vi "MESADCSubmitTestData.vi"(1 "MES_info":T1={"工号"="2300013", "站别"="F1", "站名"="写信息", "表名称"="test", "工单号"="85255", "条码"="EC82637770B0", "路径"="", "是否连接"="", "电脑名"=""}, 5 "错误输入（无错误）":errorcluster) -> (14 "result 2":i32, 15 "message":string, 17 "布尔":bool, 19 "错误输出":errorcluster)   [LabVIEW 2014]
uses:
  MES.ctl
  MESControldll.dll
panel:
  out "errbuf":string
  out "m_paramAVal":string
  out "PointGroup 2":string
  out "PointName 2":string
  out "userid 2":string
  out "POnum 1":i32
  out "result":i32
  # "2300013"
  # "1001594"
  # "0是代表OK，-1代表NG"
  # "1001608"
  # "447BBBCDFA60"
  # "447BBBA1A0D0"
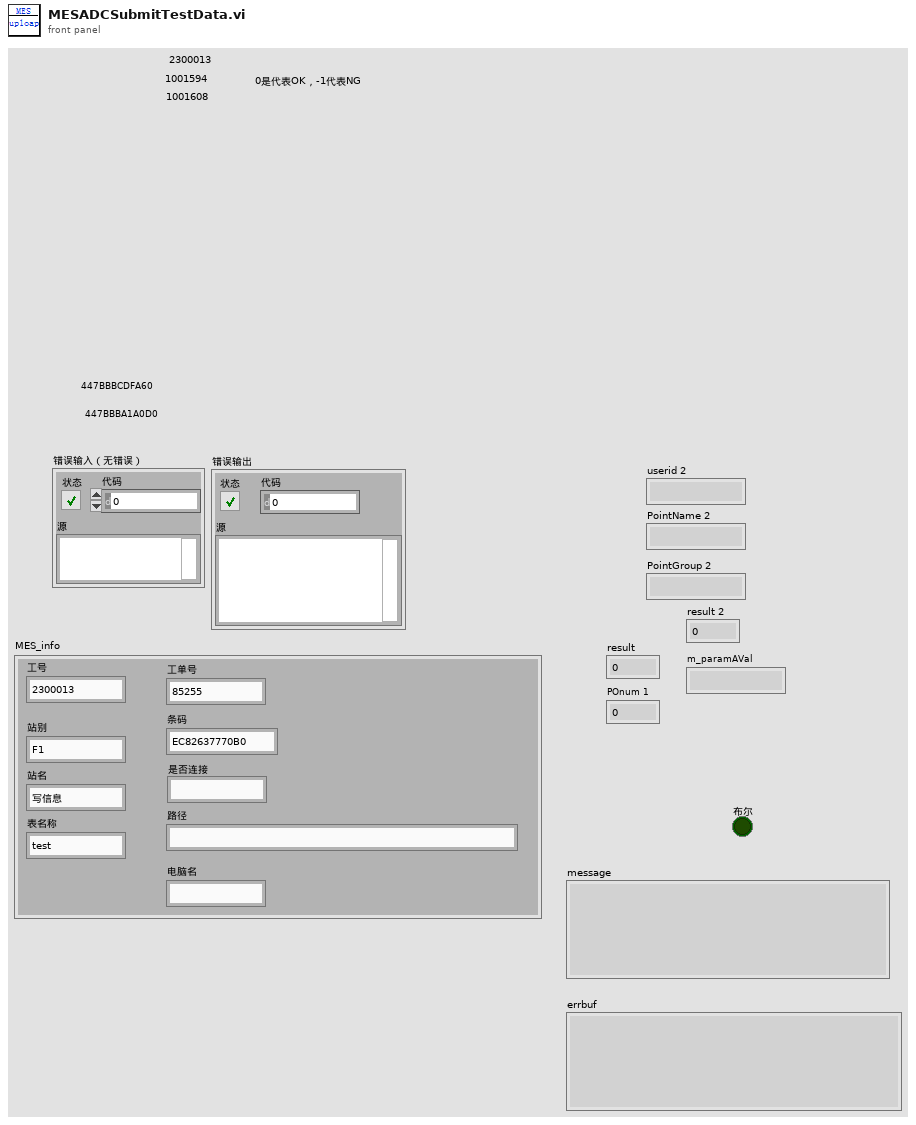
[diagram p1: front panel]
types:
  T1 = typedef "MES.ctl" = cluster{"工号":string, "站别":string, "站名":string, "表名称":string, "工单号":string, "条码":string, "路径":string, "是否连接":string, "电脑名":string}
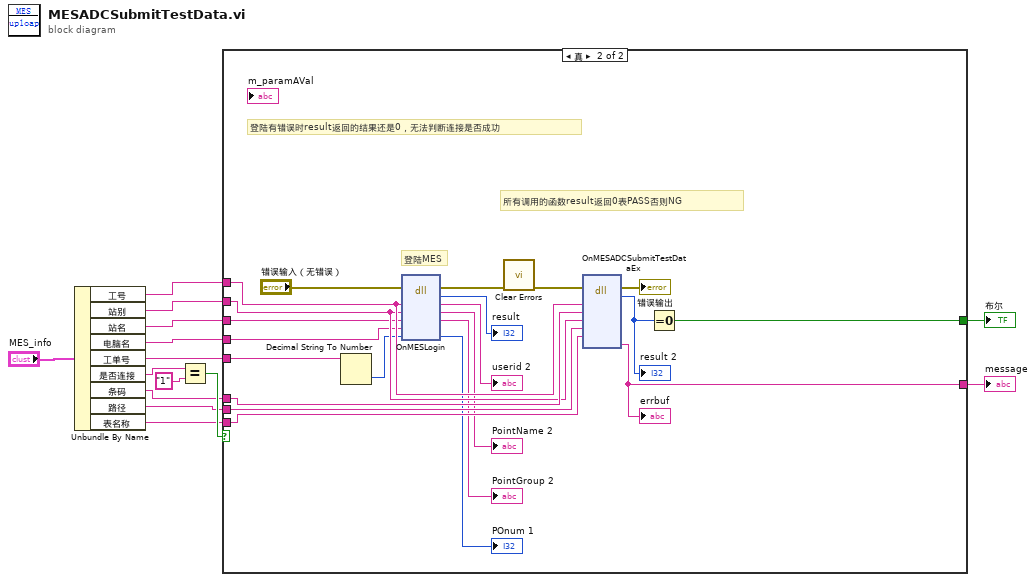
[diagram p0: block diagram]
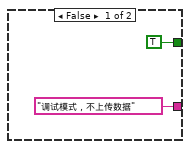
[diagram p2: hidden frame]
diagram:
  n1 = Unbundle By Name("MES_info") -> ("工号"=w1:string, "站别"=w10:string, "站名"=w9:string, "电脑名"=w8:string, "工单号"=w7:string, "是否连接"=w3:string, "条码"=w4:string, "路径"=w5:string, "表名称"=w6:string)
  n2 = Equal?(x=w3, y="1") -> (x = y?=w12:bool)
  n3 = case shown="真" w12 {
    tunnel: [TRUE w37] -> w14
    tunnel: ["调试模式，不上传数据" w36] -> w13
    tunnel: w1 -> [_ w35]
    tunnel: w4 -> [_ w34]
    tunnel: w10 -> [_ w33]
    tunnel: w7 -> [_ w32]
    tunnel: w6 -> [_ w31]
    tunnel: w9 -> [_ w30]
    tunnel: w8 -> [_ w29]
    tunnel: w5 -> [_ w28]
    frame False {
    }
    frame True {
      # "登陆MES"
      # "登陆有错误时result返回的结果还是0，无法判断连接是否成功"
      # "所有调用的函数result返回0表PASS否则NG"
      n4 = Decimal String To Number(string=w32) -> (number=w21:i32)  [unwired: 2 in, 1 out]
      n5 = dll-call lib="PTH2Dabs CUsers1001563Desktop自写吞吐量MESControldll.dll" fn="OnMESLogin"(error in="错误输入（无错误）", "userid"=w35, "PointName"=w33, "PointGroup"=w30, "PointPlace"=w29, "EquipID"=w21) -> (error out=w19:errorcluster, "result"=→"result":i32, "userid"=→"userid 2":string, "PointName"=→"PointName 2":string, "PointGroup"=→"PointGroup 2":string, "EquipID"=→"POnum 1":i32)  [unwired: 3 in, 1 out]
      n6 = call <vilib>:"Clear Errors.vi"("error in (no error)"=w19) -> ("error out"=w18:errorcluster)  [unwired: 5 in, 1 out]
      n7 = dll-call lib="PTH2Dabs CUsers1001563Desktop自写吞吐量MESControldll.dll" fn="OnMESADCSubmitTestDataEx"(error in=w18, "userid"=w35, "barcode"=w34, "pointName"=w33, "ParamAVal"=w28, "postcode"=w31) -> (error out=→"错误输出":errorcluster, "result"=w22:i32, "errbuf"=w36:string)  [unwired: 8 in, 1 out]
      "errbuf" <- w36
      "result 2" <- w22
      n8 = Equal To 0?(x=w22) -> (x = 0?=w37:bool)
    }
  }
  "布尔" <- w14
  "message" <- w13
